vi "from string.vi"(8 "error in":errorcluster, 9 "data":string, 10 "version":string, 11 "Scaling configuration in":refnum<class "Scaling configuration.lvclass">) -> (0 "error out":errorcluster, 3 "Scaling configuration out":refnum<class "Scaling configuration.lvclass">)   [LabVIEW 2013, in "Scaling configuration.lvclass"]
doc: "Provides an interface for loading a module configuration from a file or other serialized data source. It is recommended that all children of this class store data in two sets--data required for its own initialization, and any data required for parent initialization--and that each implementation uses the <b>Call Parent Method</b> primitive to de-serialize parent information. As a result, it is expected that every module configuration class calls <b>component configuration.lvclass:From String.vi</b>."
uses:
  Scaling configuration.lvclass
  <vilib>/NI/Tag Bus Module Framework/channel/TBM channel.lvclass
  controls/scale data types.ctl
  <vilib>/NI/Tag Bus Module Framework/module configuration/TBM module configuration.lvclass
  Scaling configuration.lvclass/Scaling configuration.ctl
  <vilib>/NI/Configuration Framework/serializable configuration/NISE_CEF_serializable configuration.lvclass
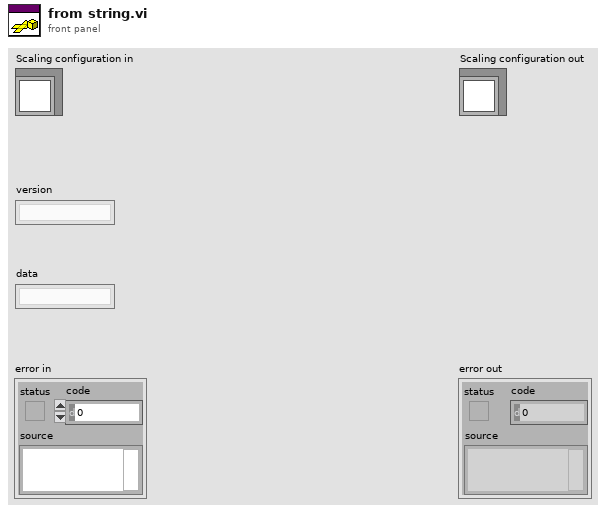
[diagram p1: front panel]
types:
  T1 = typedef "Scaling configuration.lvclass/scale data types.ctl" = enum16{"Double", "Single", "I64", "I32", "I16", "I8", "U64", "U32", "U16", "U8", "Boolean (0,1)"}
  T2 = cluster{"mappings":cluster{"input channel":refnum<class "TBM channel.lvclass">, "output channel":refnum<class "TBM channel.lvclass">, "input data type":T1, "output data type":T1}[], "name":string}[]
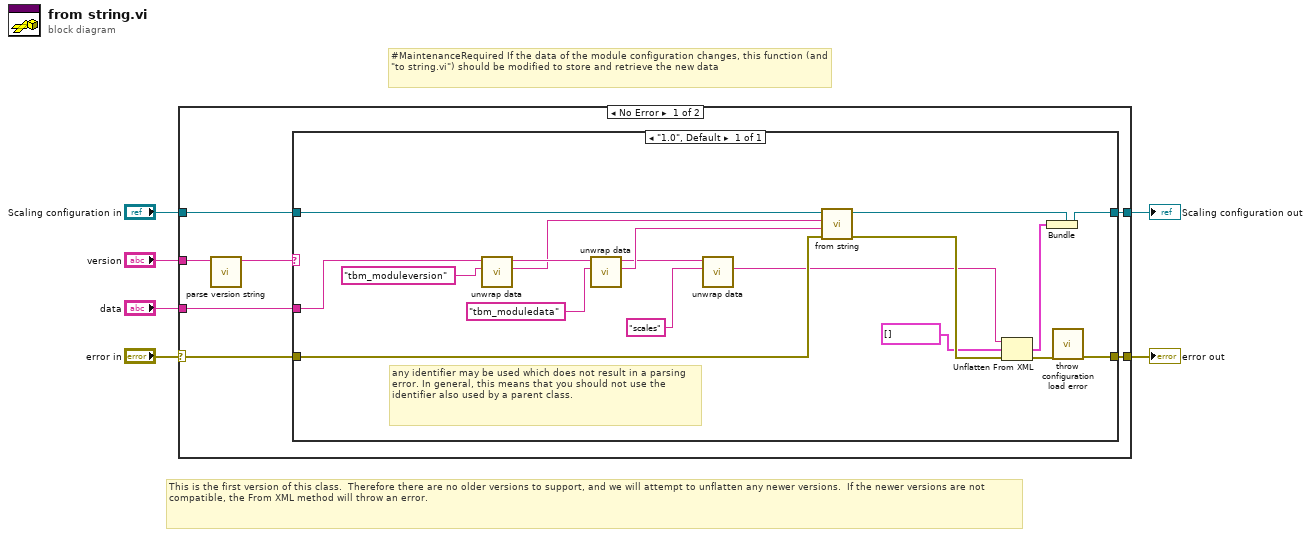
[diagram p0: block diagram]
diagram:
  # "#MaintenanceRequired If the data of the module configuration changes, this function (and \"to string.vi\") should be modified to store and retrieve the new data"
  # "This is the first version of this class.  Therefore there are no older versions to support, and we will attempt to unflatten any newer versions.  If the newer versions are not compatible, the From XML method will throw an error."
  n1 = case shown="No Error" "error in" {
    selector: "error in" -> [w7 w33]
    tunnel: "data" -> [w13 _]
    tunnel: "Scaling configuration in" -> [w12 w32]
    tunnel: [w11 w32] -> w5
    tunnel: [w10 w33] -> w4
    tunnel: "version" -> [w9 _]
    frame No Error {
      n2 = call <vilib>:"parse version string.vi"("full version"=w9) -> ("major.minor version"=w8:string)  [unwired: 7 in, 3 out]
      n3 = case shown="\"1.0\", Default" w8 {
        tunnel: w13 -> [w27]
        tunnel: w7 -> [w26]
        tunnel: w12 -> [w31]
        tunnel: [w21] -> w11
        tunnel: [w29] -> w10
        frame "1.0", Default {
          # "any identifier may be used which does not result in a parsing error. In general, this means that you should not use the identifier also used by a parent class."
          n4 = call <vilib>:"unwrap data.vi"("identifier"="tbm_moduleversion" ("additional identifier"), "data to unwrap"=w27) -> ("unwrapped data"=w22:string, "remaining string"=w28:string)  [unwired: 8 in]
          n5 = call <vilib>:"unwrap data.vi"("identifier"="tbm_moduledata" ("additional identifier"), "data to unwrap"=w28) -> ("unwrapped data"=w24:string, "remaining string"=w20:string)  [unwired: 8 in]
          n6 = call <vilib>:"unwrap data.vi"("identifier"="scales" ("additional identifier"), "data to unwrap"=w20) -> ("unwrapped data"=w15:string)  [unwired: 8 in, 1 out]
          n7 = call-parent "from string.vi"("error in"=w26, "data"=w24, "version"=w22, "module configuration in"=w31) -> ("error out"=w17:errorcluster, "module configuration out"=w30:refnum<class "Scaling configuration.lvclass">)  [unwired: 6 in]
          n8 = Unflatten From XML(xml string=w15, type=T2 [] ("scales"), error in (no error)=w17) -> (value=w14:T2, error out=w18:errorcluster)
          n9 = Bundle(cluster=w30, w14) -> (w21:refnum<class "Scaling configuration.lvclass">)
          n10 = call <vilib>:"throw configuration load error.vi"("error in"=w18) -> ("error out"=w29:errorcluster)  [unwired: 10 in]
        }
      }
    }
    frame Error {
    }
  }
  "error out" <- w4
  "Scaling configuration out" <- w5
